vi "CustomView.vi"(8 "error in":errorcluster, 10 "View Name":string, 11 "cRIO repo in":refnum<class "cRIORepo.lvclass">) -> (0 "error out":errorcluster, 3 "cRIO repo out":refnum<class "cRIORepo.lvclass">)   [LabVIEW 2013, in "cRIORepo.lvclass"]
uses:
  cRIORepo.lvclass
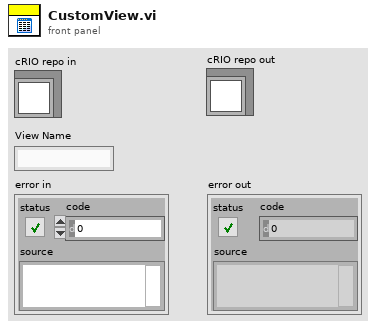
[diagram p1: front panel]
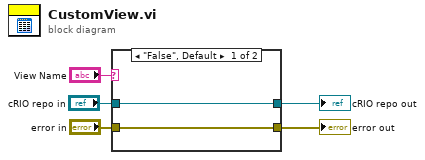
[diagram p0: block diagram]
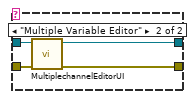
[diagram p2: hidden frame]
diagram:
  n1 = case shown="\"False\", Default" "View Name" {
    tunnel: "cRIO repo in" -> [w7 w11]
    tunnel: "error in" -> [w6 w10]
    tunnel: [w6 w9] -> w3
    tunnel: [w7 w8] -> w2
    frame "False", Default {
    }
    frame "Multiple Variable Editor" {
      n2 = call "MultiplechannelEditorUI.vi"("error in"=w10, "cRIO repo in"=w11) -> ("error out"=w9:errorcluster, "cRIO repo out"=w8:refnum<class "cRIORepo.lvclass">)  [unwired: 8 in]
    }
  }
  "cRIO repo out" <- w2
  "error out" <- w3
